vi "Audio Test.vi"() -> ()   [LabVIEW 2026]
uses:
  <vilib>/DAQmx/write.llb/DAQmx Write (Analog 1D DBL 1Chan NSamp).vi
  <vilib>/DAQmx/create/channels.llb/DAQmx Create Channel (AO-Voltage-Basic).vi
  <vilib>/DAQmx/configure/timing.llb/DAQmx Timing (Sample Clock).vi
  <vilib>/DAQmx/miscellaneous.llb/DAQmx Fill In Error Info.vi
  <vilib>/measure/NI_MABase.lvlib
panel:
  in  "Frequencies":dbl[](array[slide]) scale=0.0..2000.0
  out "error out":errorcluster
  in  "rate":dbl=1000.0 format="%0.2f"
  in  "physical channels":tag
  in  "Boolean":bool
  out "Waveform Graph 2":i16[](graph)
  in  "amplitude":dbl=1.0 format="%#_13g"
  out "Waveform Graph":waveform(dbl)(graph)
  in  "sampling info":cluster{"Fs":dbl, "#s":dbl}={"Fs"=1000.0, "#s"=1000.0} {"Fs" format="%.2p"}
  in  "n":i16
  out "Waveform Chart":i16(graph)
  out "sine out":i16
  in  "frequency (periods/tick)":fxp<+,32,0>=0.0002500000409781933
  in  "stop":bool
  # "Bb\nDb\nGb\nBb\nDb"
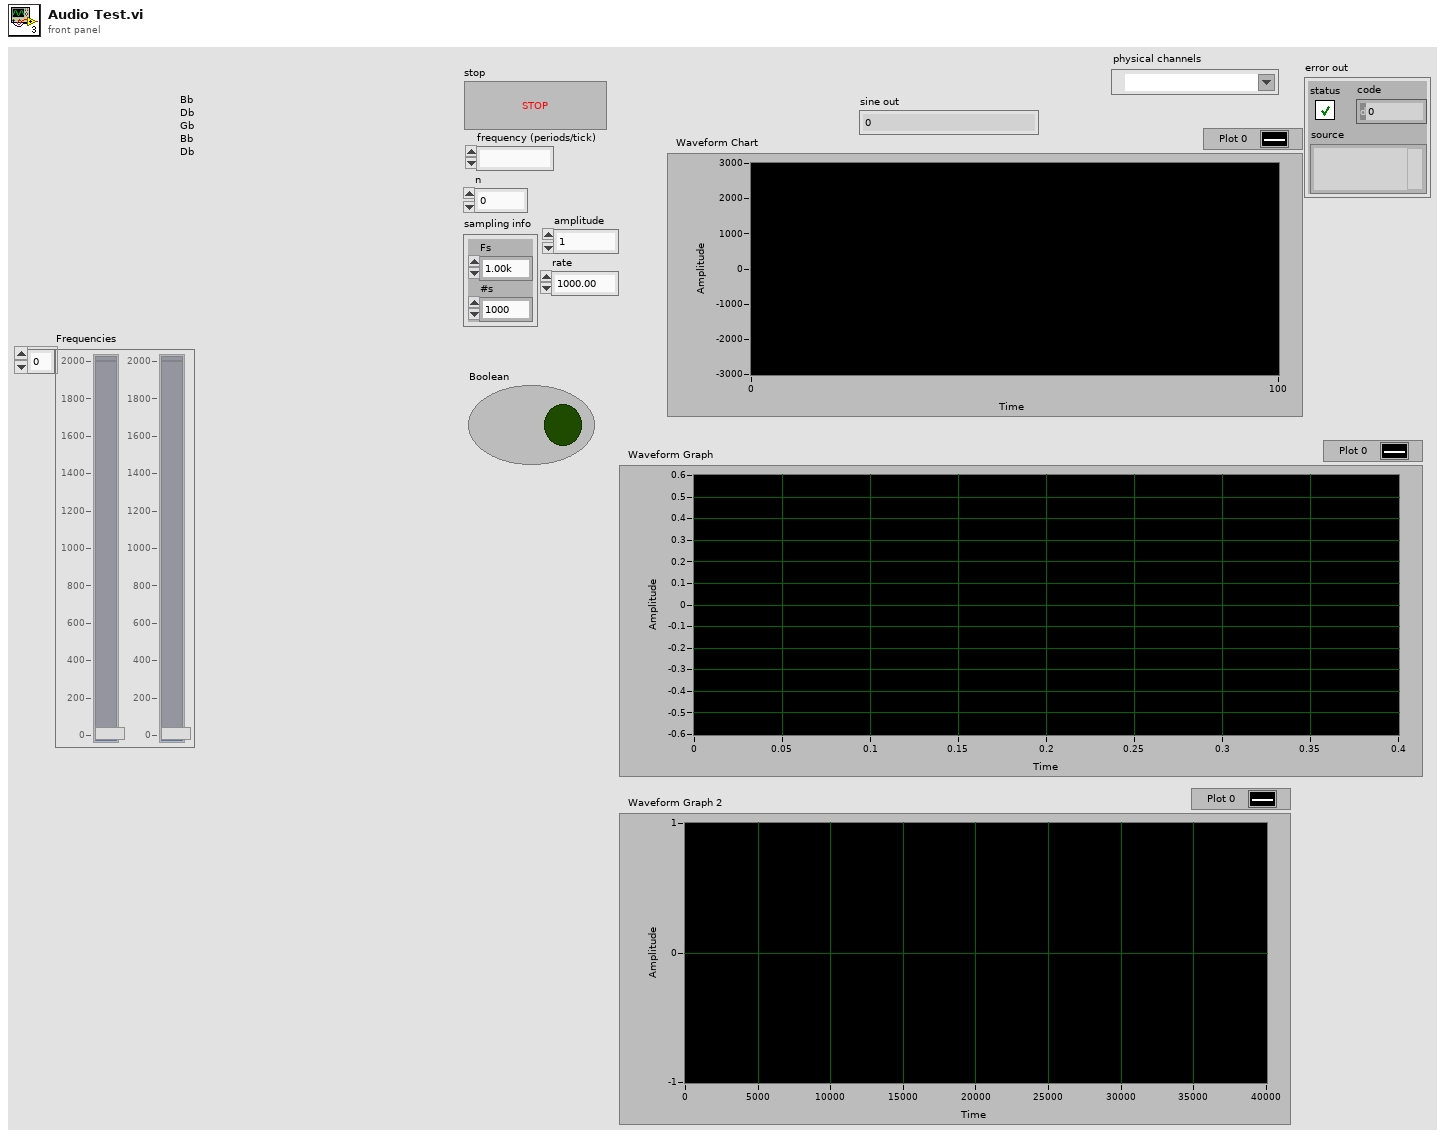
[diagram p1: front panel]
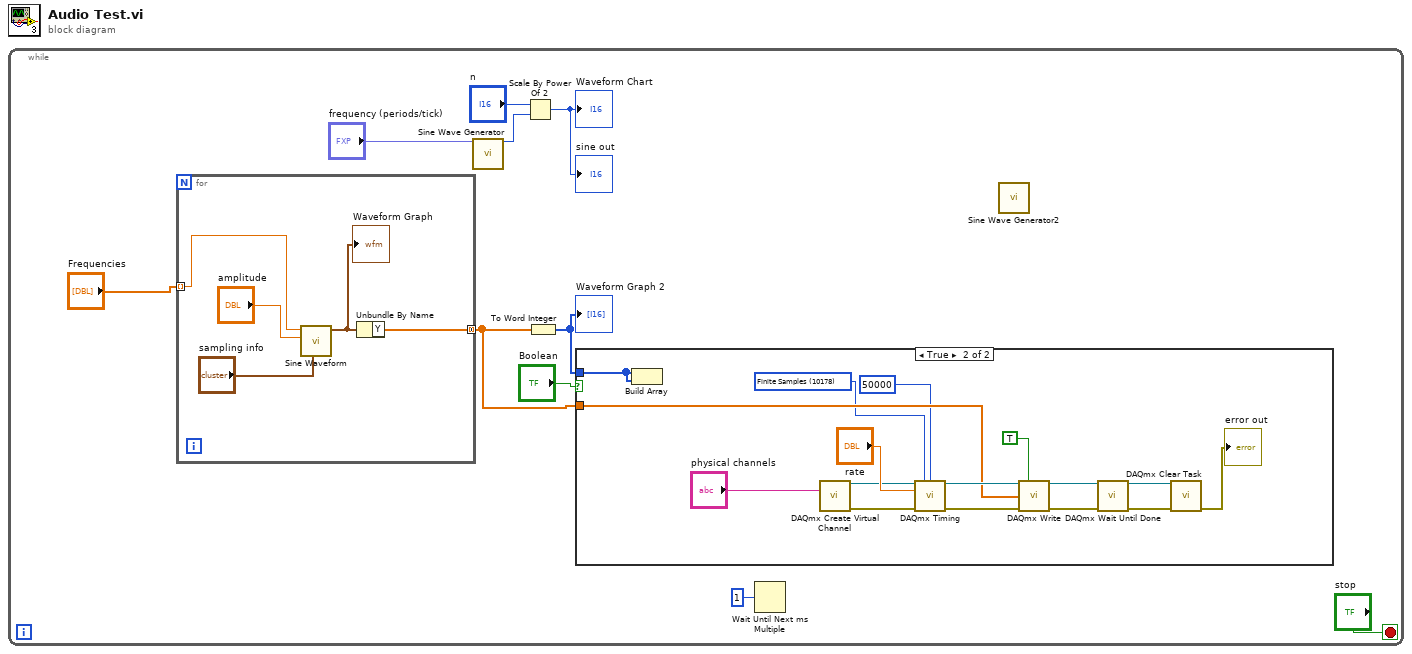
[diagram p0: block diagram]
diagram:
  n1 = while {
    stop <- "stop" stop-if-true
    n2 = for {
      tunnel: "Frequencies" -> [w11] mode=indexing
      tunnel: [w12] -> w2 mode=concatenating
      n3 = call <vilib>:"Sine Waveform.vi"("sampling info"="sampling info", "amplitude"="amplitude", "frequency"=w11) -> ("signal out"=w13:waveform(dbl))  [unwired: 7 in, 1 out]
      "Waveform Graph" <- w13
      n4 = Unbundle By Name(w13) -> ("Y"=w12:dbl[])
    }
    n5 = call "Sine Wave Generator"("frequency (periods/tick)"="frequency (periods/tick)") -> ("sine out"=w7:i16)  [unwired: 14 in]
    n6 = Scale By Power Of 2(n="n", x=w7) -> (x*2^n=→"sine out" →"Waveform Chart":i16)
    n7 = To Word Integer(number=w2) -> (16bit integer=w3:i16[])
    "Waveform Graph 2" <- w3
    n8 = case shown="True" "Boolean" {
      tunnel: w3 -> [_ w31]
      tunnel: w2 -> [_ w24]
      frame False {
      }
      frame True {
        w22 = 10178 items=["Finite Samples"=10178, "Continuous Samples"=10123, "Hardware Timed Single Point"=12522] ("sample mode")
        n9 = Build Array(w31, w31) -> ()  [unwired: 1 out]
        n10 = call-poly <vilib>:"DAQmx Create Virtual Channel.vi"("physical channels"="physical channels") -> ("task out"=w28:refnum<k21>, "error out"=w27:errorcluster)  [unwired: 13 in]
        n11 = call-poly <vilib>:"DAQmx Timing.vi"("task/channels in"=w28, "sample mode"=w22, "samples per channel"=50000, "rate"="rate", "error in"=w27) -> ("task out"=w26:refnum<k21>, "error out"=w25:errorcluster)  [unwired: 9 in]
        n12 = call-poly <vilib>:"DAQmx Write.vi"("task/channels in"=w26, "auto start"=TRUE, "data"=w24, "error in"=w25) -> ("task out"=w19:refnum<k21>, "error out"=w17:errorcluster)  [unwired: 9 in, 1 out]
        n13 = call <vilib>:"DAQmx Wait Until Done.vi"("task/channels in"=w19, "error in"=w17) -> ("task out"=w18:refnum<k21>, "error out"=w16:errorcluster)  [unwired: 12 in]
        n14 = call <vilib>:"DAQmx Clear Task.vi"("task in"=w18, "error in"=w16) -> ("error out"=→"error out":errorcluster)  [unwired: 13 in]
      }
    }
    n15 = Wait Until Next ms Multiple(millisecond multiple=u32 1) -> ()  [unwired: 1 out]
    n16 = call "Sine Wave Generator2"() -> ()  [unwired: 15 in, 1 out]
  }
